vi "Set Max Buffer Size.vi"(10 "max buffer size":u64 format="%d bytes", 11 "UDP Transceiver in":refnum<class "UDP Transceiver.lvclass">) -> (3 "UDP Transceiver out":refnum<class "UDP Transceiver.lvclass">)   [LabVIEW 2017, in "UDP Transceiver.lvlib" / "UDP Transceiver.lvclass"]
uses:
  UDP Transceiver.lvclass
  UDP Transceiver.lvclass/UDP Transceiver.ctl
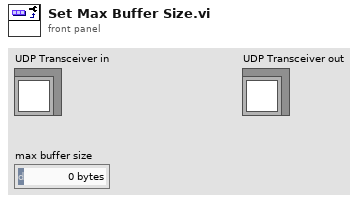
[diagram p1: front panel]
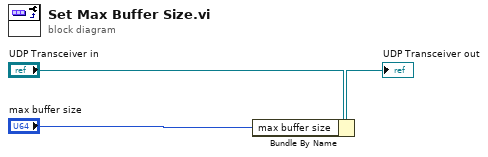
[diagram p0: block diagram]
diagram:
  n1 = Bundle By Name(cluster="UDP Transceiver in", "max buffer size"="max buffer size") -> (→"UDP Transceiver out":refnum<class "UDP Transceiver.lvclass">)
